vi "About_ANOL.vi"(8 "error in":errorcluster) -> (0 "error out":errorcluster)   [LabVIEW 2011]
panel:
  # "INL\nApplied Nano-Optics Laboratory\nPhoto-ionization Gas Sensing"
  # "www.inl.int"
  # "Written by: Pieter De Beule\nGPL license (www.gnu.org)"
  # "Click in window to continue"
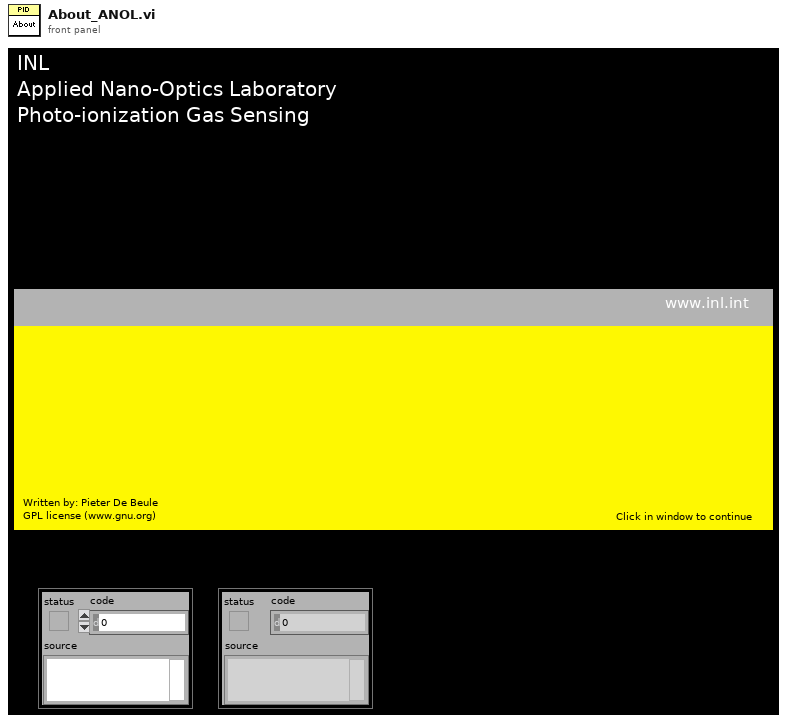
[diagram p1: front panel]
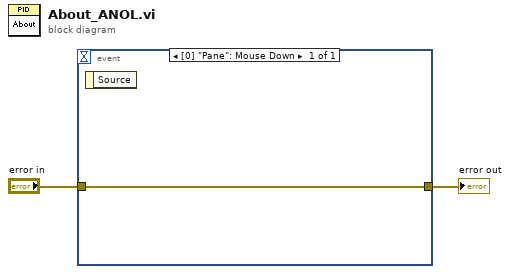
[diagram p0: block diagram]
diagram:
  n1 = event shown="[0] \"Pane\": Mouse Down" {
    selector: _ -> [_]
    dyn-events: _ -> [_]
    timeout: _ -> [_]
    tunnel: "error in" -> [w3]
    tunnel: [w3] -> w1
    event Mouse Down {
      n2 = event-data() -> ()  [unwired: 1 in, 1 out]
    }
  }
  "error out" <- w1
